vi "Zobolas Local Search Engine.vi"(6 "Scheduler":T1, 7 "Objective":T2, 8 "error in (no error)":errorcluster, 9 "Reorder?":bool, 10 "C'":u16[](array[numeric]), 11 "OSSP_Problem In":refnum<class "OSSP_Problem.lvclass">) -> (0 "error out":errorcluster, 1 "Tardiness of C\"":u16, 2 "C\"":u16[](array[numeric]), 3 "OSSP_Problem out":refnum<class "OSSP_Problem.lvclass">)   [LabVIEW 2013]
uses:
  GA/Controls/Objective.ctl
  Classes/OSSP_Problem.lvclass
  GA/Controls/Scheduler Type.ctl
  Classes/OSSP_Problem.lvclass/OSSP_Problem.ctl
  GA/SubVIS/Remove Duplicates In Array.vi
  Classes/Scheduler_Class/NonDelay Scheduler/Non Delay Scheduler Engine.vi
  Classes/OSSP_Problem_Class/Getters/Read Number of Jobs.vi
  Classes/OSSP_Problem_Class/Getters/Read Number of Machines.vi
  Classes/OSSP_Problem_Class/Getters/Read Processing Times.vi
  GA/SubVIS/Calcualte General Tardiness.vi
  Classes/OSSP_Problem_Class/Getters/Read Due Dates.vi
  Classes/Scheduler_Class/Giffler Thompson Active Schedule Engine.vi
  Classes/Scheduler_Class/Prins FIFO Scheduler Methods and Controls/Prins FIFO Scheduler.vi
  Classes/Scheduler_Class/Prins FIFO Scheduler Methods and Controls/Methods/Calculate Final Completion Times of Jobs.vi
  Classes/Scheduler_Class/Prins FIFO Scheduler Methods and Controls/Methods/Reorder Schedule(Prins FIFO) based on Start Times.vi
  Classes/Scheduler_Class/Operation to Machine Job Tuple.vi
  Classes/Scheduler_Class/Prins FIFO Scheduler Methods and Controls/Methods/UpdateMachineGaps.vi
  Classes/Scheduler_Class/Prins FIFO Scheduler Methods and Controls/Methods/UpdateJobGaps.vi
  Classes/Scheduler_Class/Prins FIFO Scheduler Methods and Controls/Methods/Find Intersecting Gaps.vi
  Classes/Scheduler_Class/Prins FIFO Scheduler Methods and Controls/Methods/Transform to Plain Job and Machine Gaps Array.vi
  Classes/Scheduler_Class/GT Algorithm Find M_ok and J_ok.vi
  Classes/Scheduler_Class/Semiactive Scheduler/Semi Active Scheduler Engine.vi
  Classes/Scheduler.lvclass
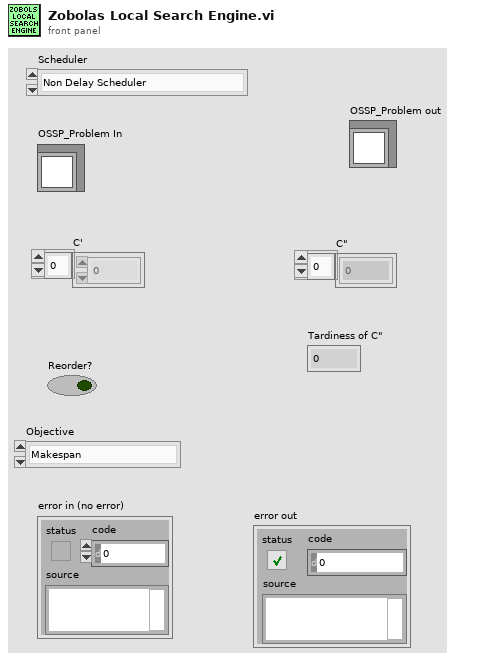
[diagram p1: front panel]
types:
  T1 = typedef "Scheduler Type.ctl" = enum16{"Non Delay Scheduler", "GT Active Scheduler", "My Faulty Scheduler", "Prins FIFO Scheduler", "SemiActive Scheduler"}
  T2 = typedef "Objective.ctl" = enum16{"Makespan", "Total Tardiness"}
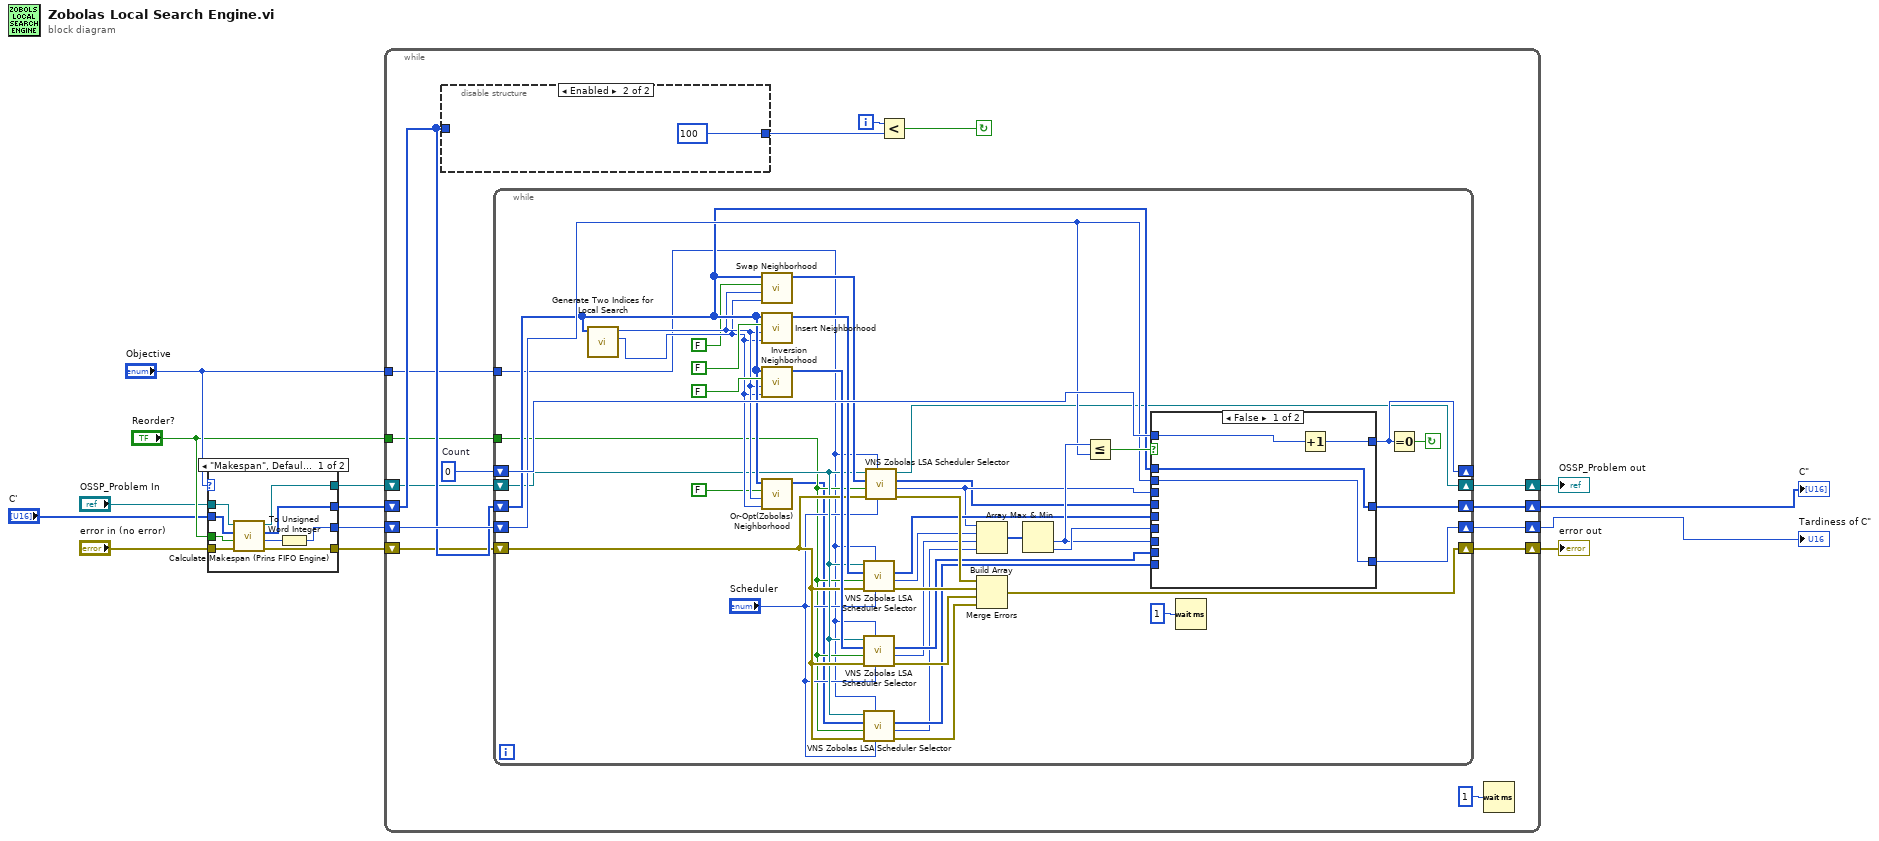
[diagram p0: block diagram]
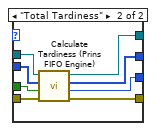
[diagram p2: hidden frame]
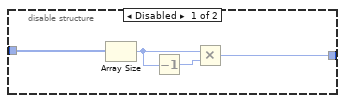
[diagram p3: hidden frame]
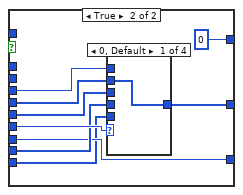
[diagram p4: hidden frame]
diagram:
  n1 = case shown="\"Makespan\", Default" "Objective" {
    tunnel: "C'" -> [w15 w24]
    tunnel: [w22 w28] -> w11
    tunnel: "Reorder?" -> [w16 w23]
    tunnel: [w21 w30] -> w7
    tunnel: "OSSP_Problem In" -> [w19 w29]
    tunnel: [w18 w27] -> w5
    tunnel: "error in (no error)" -> [w17 w26]
    tunnel: [w14 w25] -> w3
    frame "Makespan", Default {
      n2 = call "Calculate Makespan (Prins FIFO Engine).vi"("error in (no error)"=w17, "Reorder?"=w16, "Schedule In"=w15, "OSSP_Problem in"=w19) -> ("error out"=w14:errorcluster, "Makespan"=w20:i32, "Schedule Out"=w21:u16[], "OSSP_Problem out"=w18:refnum<class "OSSP_Problem.lvclass">)  [unwired: 4 in]
      n3 = To Unsigned Word Integer(number=w20) -> (unsigned 16bit integer=w22:u16)
    }
    frame "Total Tardiness" {
      n4 = call "Calculate Tardiness (Prins FIFO Engine).vi"("error in (no error)"=w26, "Reorder?"=w23, "Schedule In"=w24, "OSSP_Problem in"=w29) -> ("error out"=w25:errorcluster, "Tardiness(Prins FIFO Engine)"=w28:u16, "Schedule Out"=w30:u16[], "OSSP_Problem out"=w27:refnum<class "OSSP_Problem.lvclass">)  [unwired: 3 in, 1 out]
    }
  }
  n5 = while {
    shift-right: [w43] -> w13
    shift-left: w7 -> [w41]
    shift-right: [w42] -> w12
    shift-left: w11 -> [w45]
    tunnel: "Objective" -> [w36]
    tunnel: "Reorder?" -> [w35]
    shift-right: [w32] -> w2
    shift-left: w5 -> [w34]
    shift-right: [w31] -> w1
    shift-left: w3 -> [w33]
    i -> [w40]
    stop <- w38 continue-if-true
    w44 = 0  # Count
    n6 = disable-structure shown="Enabled" {
      disable-tunnel: w41 -> [w49 _]
      disable-tunnel: [w46 100] -> w39
      frame Disabled {
        n7 = Array Size(array=w49) -> (size(s)=w48:i32)
        n8 = Decrement(x=w48) -> (x-1=w47:i32)
        n9 = Multiply(x=w48, y=w47) -> (x*y=w46:i32)
      }
      frame Enabled {
      }
    }
    n10 = while {
      shift-right: [w86] -> w43
      shift-left: w41 -> [w79]
      shift-right: [w81] -> _
      shift-left: w44 -> [w85]
      shift-right: [w83] -> w42
      shift-left: w45 -> [w82]
      tunnel: w36 -> [w55]
      tunnel: w35 -> [w57]
      shift-right: [w73] -> w32
      shift-left: w34 -> [w59]
      shift-right: [w71] -> w31
      shift-left: w33 -> [w61]
      stop <- w80 continue-if-true
      n11 = call "Generate Two Indices for Local Search.vi"("Schedule in"=w79) -> ("w"=w77:i32, "y"=w78:i32)  [unwired: 9 in]
      n12 = call "Swap Neighborhood.vi"("w"=w77, "y"=w78, "Generate Random Indices?"=FALSE, "Schedule In"=w79) -> ("Schedule Out"=w70:u16[])  [unwired: 7 in]
      n13 = call "Insert Neighborhood.vi"("w"=w77, "y"=w78, "Generate Random Indices?"=FALSE, "C'"=w79) -> ("Chromosome Out"=w69:u16[])  [unwired: 7 in]
      n14 = call "Inversion Neighborhood.vi"("w"=w77, "y"=w78, "Generate Random Indices?"=FALSE, "Schedule in"=w79) -> ("Schedule out"=w65:u16[])  [unwired: 7 in]
      n15 = call "Or-Opt(Zobolas) Neighborhood.vi"("w"=w77, "y"=w78, "Generate Random Indices?"=FALSE, "C'"=w79) -> ("Chromosome Out"=w56:u16[])  [unwired: 7 in]
      n16 = call "VNS Zobolas LSA Scheduler Selector.vi"("Scheduler"="Scheduler", "Objective"=w55, "error in (no error)"=w61, "Reorder?"=w57, "Schedule in"=w69, "OSSP_Problem in"=w59) -> ("error out"=w67:errorcluster, "Total Tardiness (U16)"=w66:u16, "Schedule out"=w68:u16[])  [unwired: 2 in, 1 out]
      n17 = call "VNS Zobolas LSA Scheduler Selector.vi"("Scheduler"="Scheduler", "Objective"=w55, "error in (no error)"=w61, "Reorder?"=w57, "Schedule in"=w65, "OSSP_Problem in"=w59) -> ("error out"=w63:errorcluster, "Total Tardiness (U16)"=w62:u16, "Schedule out"=w64:u16[])  [unwired: 2 in, 1 out]
      n18 = call "VNS Zobolas LSA Scheduler Selector.vi"("Scheduler"="Scheduler", "Objective"=w55, "error in (no error)"=w61, "Reorder?"=w57, "Schedule in"=w56, "OSSP_Problem in"=w59) -> ("error out"=w60:errorcluster, "Total Tardiness (U16)"=w53:u16, "Schedule out"=w54:u16[])  [unwired: 2 in, 1 out]
      n19 = call "VNS Zobolas LSA Scheduler Selector.vi"("Scheduler"="Scheduler", "Objective"=w55, "error in (no error)"=w61, "Reorder?"=w57, "Schedule in"=w70, "OSSP_Problem in"=w59) -> ("error out"=w72:errorcluster, "Total Tardiness (U16)"=w52:u16, "Schedule out"=w51:u16[], "OSSP_Problem out"=w73:refnum<class "OSSP_Problem.lvclass">)  [unwired: 2 in]
      n20 = Build Array(w52, w66, w62, w53) -> (w89:u16[])
      n21 = Merge Errors(w72, w67, w63, w60) -> (w71:errorcluster)
      n22 = Array Max & Min(array=w89) -> (min value=w84:u16, min index (indices)=w87:i32)  [unwired: 2 out]
      n23 = Less Or Equal?(x=w84, y=w82) -> (x <= y?=w88:bool)
      n24 = case shown="False" w88 {
        tunnel: w87 -> [_ w104]
        tunnel: w52 -> [_ w103]
        tunnel: [w95 w102] -> w86
        tunnel: w79 -> [w95 _]
        tunnel: w68 -> [_ w101]
        tunnel: w64 -> [_ w100]
        tunnel: w85 -> [w94 _]
        tunnel: [w93 0] -> w81
        tunnel: [w92 w98] -> w83
        tunnel: w84 -> [_ w98]
        tunnel: w82 -> [w92 _]
        tunnel: w54 -> [_ w97]
        tunnel: w51 -> [_ w96]
        frame False {
          n25 = Increment(x=w94) -> (x+1=w93:i32)
        }
        frame True {
          n26 = case shown="0, Default" w104 {
            tunnel: w103 -> [_ _ _ _]
            tunnel: [w105 w106 w107 w108] -> w102
            tunnel: w101 -> [_ w106 _ _]
            tunnel: w100 -> [_ _ w107 _]
            tunnel: w97 -> [_ _ _ w108]
            tunnel: w96 -> [w105 _ _ _]
            frame 0, Default {
            }
            frame 1 {
            }
            frame 2 {
            }
            frame 3 {
            }
          }
        }
      }
      n27 = Wait (ms)(milliseconds to wait=u32 1) -> ()  [unwired: 1 out]
      n28 = Equal To 0?(x=w81) -> (x = 0?=w80:bool)
    }
    n29 = Less?(x=w40, y=w39) -> (x < y?=w38:bool)
    n30 = Wait (ms)(milliseconds to wait=u32 1) -> ()  [unwired: 1 out]
  }
  "C\"" <- w13
  "Tardiness of C\"" <- w12
  "OSSP_Problem out" <- w2
  "error out" <- w1
